vi "Sigmoid.vi"(2 "Z":dbl[][](array[numeric])) -> (0 "Sigmoid(Z)":dbl[][](array[numeric]))   [LabVIEW 2020]
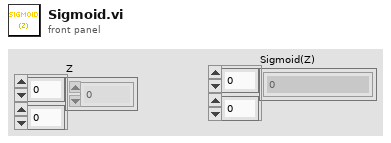
[diagram p1: front panel]
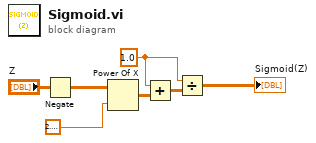
[diagram p0: block diagram]
diagram:
  w6 = 1.0 ("x")
  n1 = Negate(x="Z") -> (-x=w3:dbl[][])
  n2 = Power Of X(1:2.718281828459045, 2:w3) -> (0:w1:dbl[][])
  n3 = Add(x=w6, y=w1) -> (x+y=w5:dbl[][])
  n4 = Divide(x=w6, y=w5) -> (x/y=→"Sigmoid(Z)":dbl[][])
